vi "Read Misc Settings.vi"(4 "Reload":bool, 5 "error in (no error)":errorcluster, 6 "Key":string, 7 "Section":string, 8 "DB_ADO in":refnum<class "Config Data_DB_ADO.lvclass">) -> (0 "error out":errorcluster, 2 "p_value":string, 3 "DB_ADO out":refnum<class "Config Data_DB_ADO.lvclass">)   [LabVIEW 2020, in "Config Data.lvlib" / "Config Data_DB_ADO.lvclass"]
uses:
  Config Data_DB_ADO.lvclass
  toolbox/ADO Database Drivers/ADO Database Drivers.lvlib
  Config Data_DB.lvclass
  C:/Users/Fred Guo/Desktop/Release 19/_libraries/Config Data/DB/Config Data_DB.lvclass
  C:/Users/Fred Guo/Desktop/Release 19/_libraries/Config Data/Config Data.lvclass
  C:/Users/Fred Guo/Desktop/Release 19/_libraries/Config Data/DB/ADO/Config Data_DB_ADO.lvclass
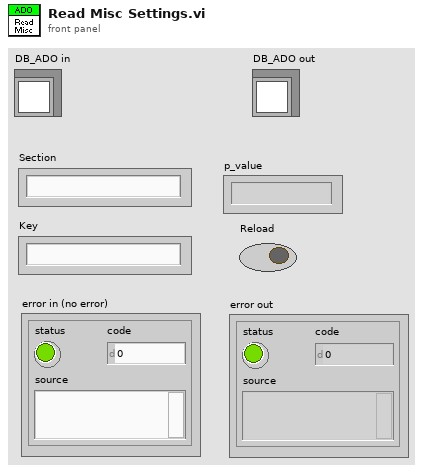
[diagram p1: front panel]
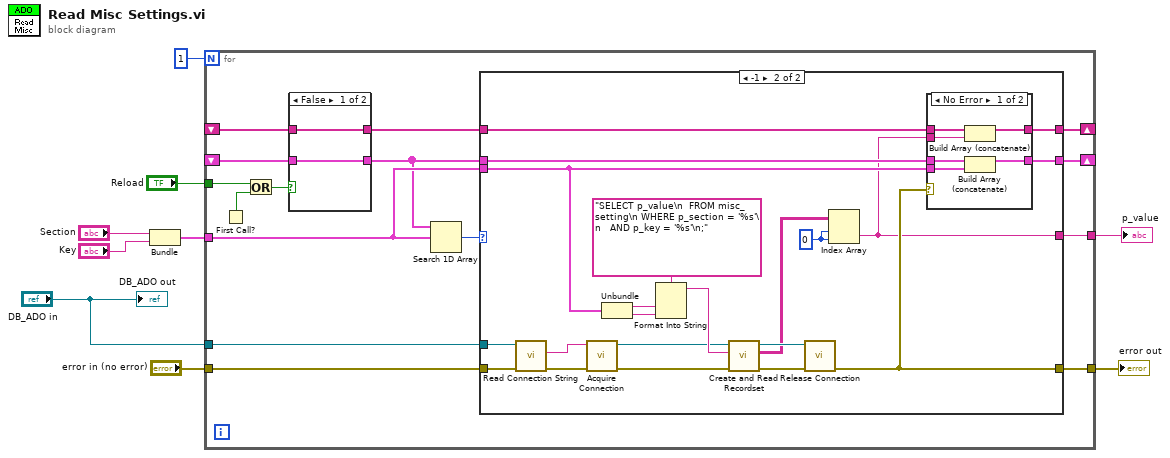
[diagram p0: block diagram]
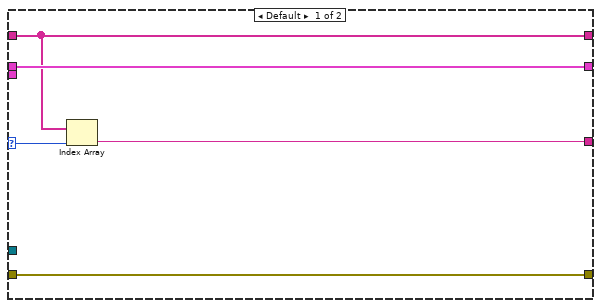
[diagram p3: hidden frame]
diagram:
  n1 = Bundle("Section"="Section", "Key"="Key") -> (w9:cluster{"Section":string, "Key":string})  [unwired: 1 in]
  n2 = for {
    N: 1 -> [_]
    tunnel: "error in (no error)" -> [w24]
    tunnel: [w23] -> w3
    shift-right: [w22] -> _
    shift-left: _ -> [w17]
    shift-right: [w21] -> _
    shift-left: _ -> [w16]
    tunnel: w9 -> [w19]
    tunnel: [w13] -> w4
    tunnel: "DB_ADO in" -> [w12]
    tunnel: "Reload" -> [w10]
    n3 = First Call?() -> (First Call?: T/F=w18:bool)
    n4 = Or(x=w10, y=w18) -> (x .or. y?=w11:bool)
    n5 = case shown="False" w11 {
      tunnel: w17 -> [w26 _]
      tunnel: w16 -> [w25 _]
      tunnel: [w26 _] -> w15
      tunnel: [w25 _] -> w14
      frame False {
      }
      frame True {
      }
    }
    n6 = Search 1D Array(1D array=w14, element=w19) -> (index of element=w20:i32)  [unwired: 1 in]
    n7 = case shown="-1" w20 {
      selector: w20 -> [w29 _]
      tunnel: w24 -> [w31 w34]
      tunnel: [w31 w45] -> w23
      tunnel: w15 -> [w28 w44]
      tunnel: [w28 w42] -> w22
      tunnel: [w30 w41] -> w21
      tunnel: w14 -> [w30 w43]
      tunnel: w19 -> [_ w38]
      tunnel: [w27 w37] -> w13
      tunnel: w12 -> [_ w35]
      frame Default {
        n8 = Index Array(array=w28, index=w29) -> (element=w27:string)
      }
      frame -1 {
        w46 = 0 ("disabled index (col)")
        n9 = call "Read Connection String.vi"("Error In"=w34, "DB In"=w35) -> ("Error Out"=w36:errorcluster, "Connection String"=w52:string)  [unwired: 3 in, 1 out]
        n10 = call "Acquire Connection.vi"("error in (no error)"=w36, "Connection String"=w52) -> ("error out"=w32:errorcluster, "Connection"=w33:refnum<k7>)  [unwired: 3 in, 1 out]
        n11 = Unbundle(w38) -> ("Section"=w40:string, "Key"=w39:string)
        n12 = Format Into String(format string="SELECT p_value\n  FROM misc_setting\n WHERE p_section = '%s'\n   AND p_key = '%s'\n;", w40, w39) -> (resulting string=w48:string)  [unwired: 2 in, 1 out]
        n13 = call "Create and Read Recordset.vi"("error in (no error)"=w32, "Source"=w48, "Connection In"=w33) -> ("error out"=w51:errorcluster, "DB Data"=w49:string[][], "Connection Out"=w50:refnum<k7>)  [unwired: 2 in, 2 out]
        n14 = call "Release Connection.vi"("error in"=w51, "Connection"=w50) -> ("error out"=w45:errorcluster)  [unwired: 5 in]
        n15 = Index Array(array=w49, index (row)=w46, index (col)=w46) -> (element=w37:string)
        n16 = case shown="No Error" w45 {
          tunnel: w44 -> [w58 w60]
          tunnel: w43 -> [w55 w59]
          tunnel: [w56 w60] -> w42
          tunnel: [w54 w59] -> w41
          tunnel: w37 -> [w57 _]
          tunnel: w38 -> [w53 _]
          frame No Error {
            n17 = Build Array (concatenate)(w58, w57) -> (w56:string[])
            n18 = Build Array (concatenate)(w55, w53) -> (w54:cluster{"Section":string, "Key":string}[])
          }
          frame Error {
          }
        }
      }
    }
  }
  "p_value" <- w4
  "error out" <- w3
  "DB_ADO out" <- "DB_ADO in"
